vi "clear Session Data.vi"(0 "Session in":refnum<class "Engine.lvclass">, 11 "error in":errorcluster) -> (4 "Session out":refnum<class "Engine.lvclass">, 15 "error out":errorcluster)   [LabVIEW 2020, in "HTS.lvlib" / "Engine.lvclass"]
uses:
  Engine.lvclass
  Engine.lvclass/Engine.ctl
  <userlib>/_Session Fwk/Session - Root.lvclass
  VariableContainer/VariableContainer.lvclass
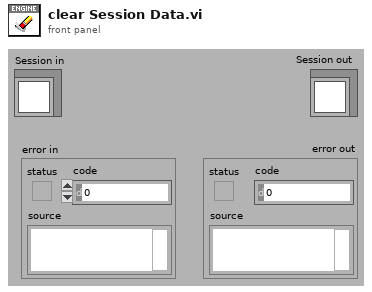
[diagram p1: front panel]
types:
  T1 = typedef "HTS.lvlib/VariableContainer.lvclass/Session Handle.ctl" = refnum<data-value>
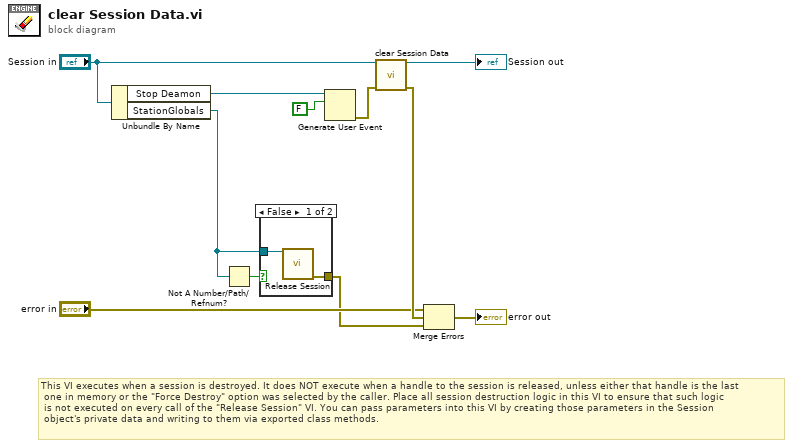
[diagram p0: block diagram]
diagram:
  # "This VI executes when a session is destroyed. It does NOT execute when a handle to the session is released, unless either that handle is the last\n one in memory or the \"Force Destroy\" option was selected by the caller. Place all session destruction logic in this VI to ensure that such logic\n is not executed on every call of the \"Release Session\" VI. You can pass parameters into this VI by creating those parameters in the Session \n object's private data and writing to them via exported class methods."
  n1 = Unbundle By Name("Session in") -> ("Stop Deamon"=w10:refnum<user-event>, "StationGlobals"=w2:T1)
  n2 = Not A Number/Path/Refnum?(number/path/refnum=w2) -> (NaN/Path/Refnum?=w3:bool)
  n3 = case shown="False" w3 {
    tunnel: w2 -> [w13 _]
    tunnel: [w12 _] -> w1
    frame False {
      n4 = call "Release Session.vi"("Session Handle"=w13) -> ("error out"=w12:errorcluster)  [unwired: 14 in]
    }
    frame True {
    }
  }
  n5 = Generate User Event(user event=w10, event data cluster=FALSE ("event data")) -> (error out=w8:errorcluster)  [unwired: 2 in, 1 out]
  n6 = call-parent "clear Session Data.vi"("OBJ - Measurement Session in"="Session in", "error in"=w8) -> ("OBJ - Measurement Session out"=→"Session out":refnum<class "Engine.lvclass">, "error out"=w11:errorcluster)  [unwired: 12 in]
  n7 = Merge Errors("error in", w11, w1) -> (→"error out":errorcluster)
